vi "SetConfig.vi"(8 "error in (no error)":errorcluster, 10 "Variant":variant, 11 "MultiBandState in":refnum<class "MultiBandState.lvclass">) -> (0 "error out":errorcluster, 3 "MultiBandState out":refnum<class "MultiBandState.lvclass">)   [LabVIEW 2014, in "Functions.lvlib" / "MultiBandState.lvclass"]
uses:
  MultiBandState.lvclass
  FunctionBaseClass/FunctionBase.lvclass
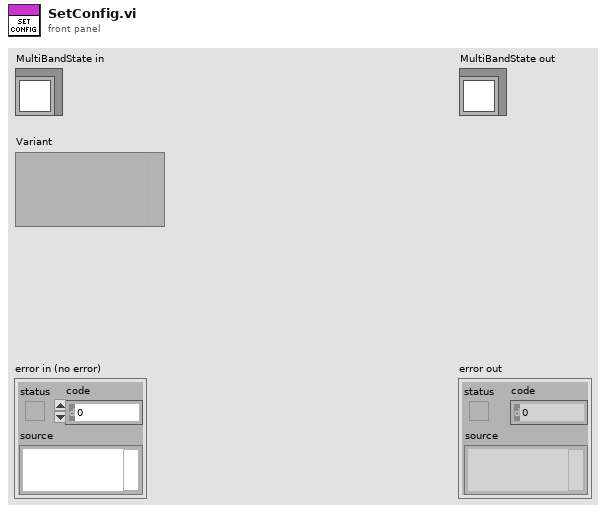
[diagram p1: front panel]
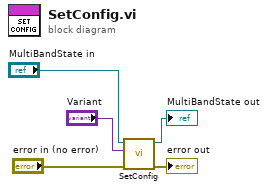
[diagram p0: block diagram]
diagram:
  n1 = call-parent "SetConfig.vi"("error in (no error)"="error in (no error)", "Variant"="Variant", "FunctionBase in"="MultiBandState in") -> ("error out"=→"error out":errorcluster, "FunctionBase out"=→"MultiBandState out":refnum<class "MultiBandState.lvclass">)  [unwired: 7 in]
